vi "Compile Res Sim.vi"(8 "error in (no error)":errorcluster, 10 "SLSC Compiled in":T1 {"FIU Engine Data"."Ordered Fault Channels" format="%.0x"; "FIU Engine Data"."FIU IDs"."Slot #" max=15; "FIU Engine Data"."FIU IDs"."Chip Address (A2 A1 A0)" max=7}, 11 "Device Item Ref in":T7 format="%.0x") -> (0 "error out":errorcluster, 2 "SLSC Compiled out":T1 {"FIU Engine Data"."Ordered Fault Channels" format="%.0x"; "FIU Engine Data"."FIU IDs"."Slot #" max=15; "FIU Engine Data"."FIU IDs"."Chip Address (A2 A1 A0)" max=7}, 3 "Device Item Ref out":T7 format="%.0x")   [LabVIEW 2014, in "SLSC configuration System Explorer.lvlib"]
uses:
  SLSC configuration System Explorer.lvlib
  <vilib>/NI Veristand/Custom Device API/Custom Device Item Ref.ctl
  Shared/SLSC compiled.ctl
  Shared/Res Sim compiled.ctl
  Shared/Type Defs/FIU Engine Data.ctl
  Shared/Type Defs/FIU IDs.ctl
  Example/SPI Utility/Slot #.ctl
  Example/MCP23S17/Chip Address.ctl
  Shared/Card Postion.ctl
  <vilib>/NI Veristand/Custom Device API/Data Access Type.ctl
  Shared/Constants.vi
  <vilib>/NI Veristand/Custom Device API/Get Item Property (Variant).vi
  <vilib>/NI Veristand/Custom Device API/Get Item Property (U16).vi
  <vilib>/NI Veristand/Custom Device Tools/Custom Device Utility Library/Custom Device Utility Library.lvlib
  Shared/SLSC configuration Shared.lvlib
  <vilib>/NI Veristand/Custom Device API/Custom Device API.lvlib
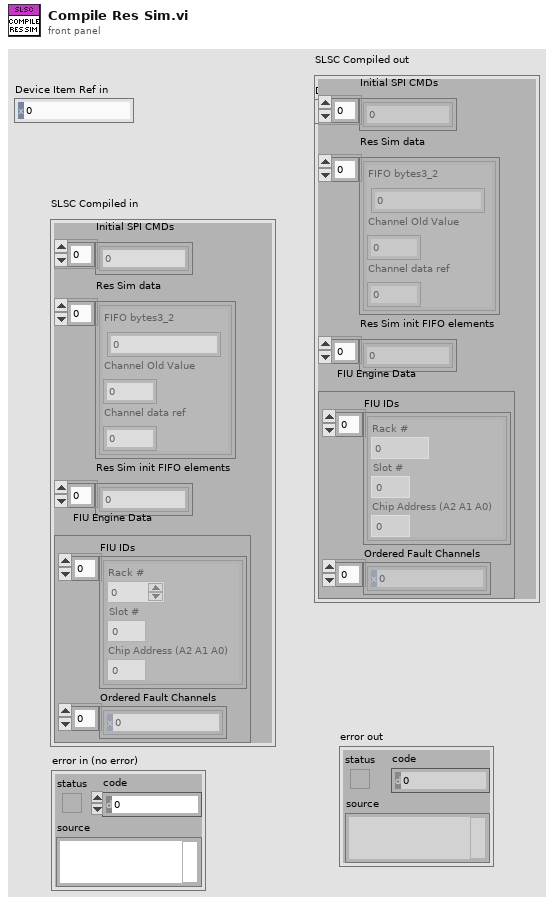
[diagram p1: front panel]
types:
  T1 = typedef "SLSC configuration Shared.lvlib/SLSC compiled.ctl" = cluster{"Initial SPI CMDs":u64[], "Res Sim data ":T2[], "Res Sim init FIFO elements":u32[], "FIU Engine Data":T3}
  T2 = typedef "SLSC configuration Shared.lvlib/Res Sim compiled.ctl" = cluster{"FIFO bytes3_2":u16, "Channel Old Value":dbl, "Channel data ref":i32}
  T3 = typedef "SLSC configuration Shared.lvlib/FIU Engine Data.ctl" = cluster{"FIU IDs":T4[], "Ordered Fault Channels":T7[]}
  T4 = typedef "SLSC configuration Shared.lvlib/FIU IDs.ctl" = cluster{"Rack #":u8, "Slot #":T5, "Chip Address (A2 A1 A0)":T6}
  T5 = typedef "SLSC configuration Shared.lvlib/Slot #.ctl" = u8
  T6 = typedef "SLSC configuration Shared.lvlib/Chip Address.ctl" = u8
  T7 = typedef "Custom Device API.lvlib/Custom Device Item Ref.ctl" = u64
  T8 = typedef "SLSC configuration Shared.lvlib/Card Postion.ctl" = cluster{"Chassis #":u8, "Slot #":u8}
  T9 = typedef "Custom Device API.lvlib/Data Access Type.ctl" = enum16{"Read", "Write"}
  T10 = typedef "Custom Device API.lvlib/Custom Device Channel.ctl" = cluster{"Type":T11, "Units":string, "Default Value":dbl, "Faultable":bool, "Scalable":bool}
  T11 = typedef "Custom Device API.lvlib/Custom Device Channel Type.ctl" = enum16{"Input", "Output"}
  T12 = typedef "Custom Device API.lvlib/Data Reference.ctl" = i32
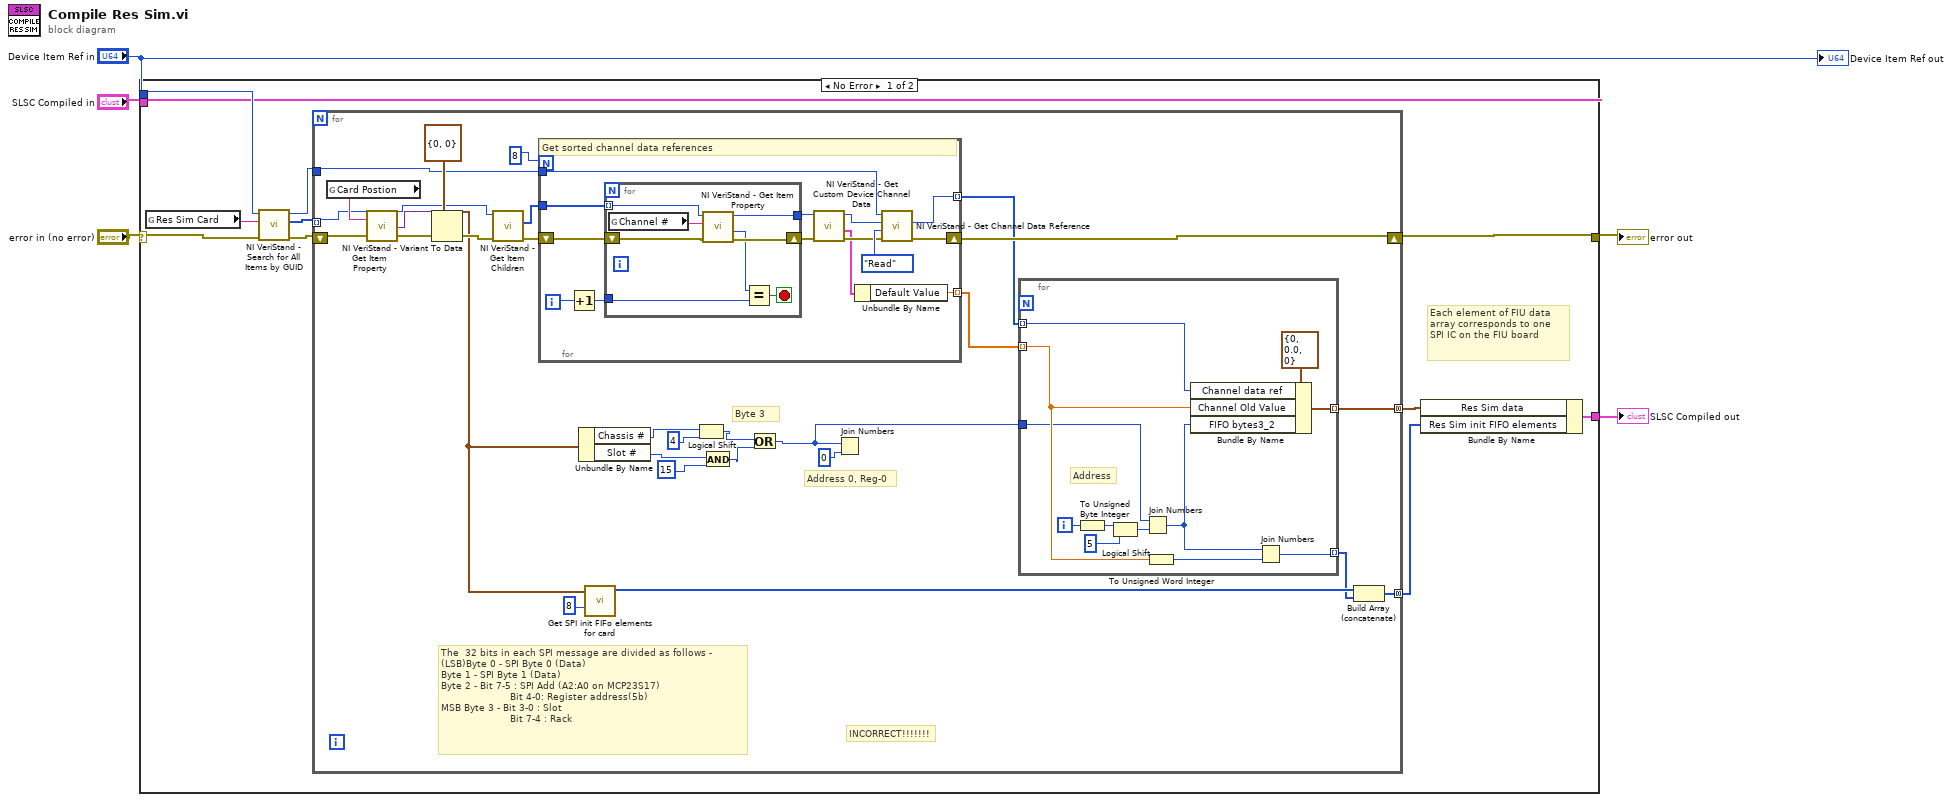
[diagram p0: block diagram]
diagram:
  n1 = case shown="No Error" "error in (no error)" {
    selector: "error in (no error)" -> [w9 w81]
    tunnel: [w12 w81] -> w5
    tunnel: "Device Item Ref in" -> [w11 _]
    tunnel: [w10 w80] -> w3
    tunnel: "SLSC Compiled in" -> [w8 w80]
    frame No Error {
      # "Each element of FIU data array corresponds to one SPI IC on the FIU board"
      n2 = global read "Constants.vi" "Res Sim Card"() -> (w16:string)
      n3 = call <vilib>:"NI VeriStand - Search for All Items by GUID.vi"("error in"=w9, "Item GUID"=w16, "Section Ref in"=w11) -> ("error out"=w15:errorcluster, "Item Refs"=w13:T7[], "Section Ref out"=w14:T7)  [unwired: 5 in, 1 out]
      n4 = for {
        tunnel: w14 -> [w29]
        tunnel: w13 -> [w31] mode=indexing
        tunnel: [w22] -> w7 mode=concatenating
        shift-right: [w24] -> w12
        shift-left: w15 -> [w39]
        tunnel: [w21] -> w6 mode=concatenating
        # "INCORRECT!!!!!!!"
        # "The  32 bits in each SPI message are divided as follows -\n(LSB)Byte 0 - SPI Byte 0 (Data)\nByte 1 - SPI Byte 1 (Data)\nByte 2 - Bit 7-5 : SPI Add (A2:A0 on MCP23S17)\n                       Bit 4-0: Register address(5b)\nMSB Byte 3 - Bit 3-0 : Slot\n                       Bit 7-4 : Rack"
        # "Address 0, Reg-0"
        # "Byte 3"
        n5 = global read "Constants.vi" "Card Postion"() -> (w38:string)
        n6 = call-poly <vilib>:"NI VeriStand - Get Item Property.vi"("error in (no error)"=w39, "Property Name"=w38, "Item Ref in"=w31) -> ("error out"=w41:errorcluster, "Value"=w42:variant, "Item Ref out"=w30:T7)  [unwired: 5 in, 1 out]
        n7 = Variant To Data(error in=w41, type=T8 {"Chassis #"=0, "Slot #"=0} ("Card Position"), Variant=w42) -> (data=w28:T8, error out=w40:errorcluster)
        n8 = call <vilib>:"NI VeriStand - Get Item Children.vi"("error in (no error)"=w40, "Item Ref in"=w30) -> ("error out"=w25:errorcluster, "Child Refs"=w44:T7[])  [unwired: 6 in, 2 out]
        n9 = for {
          N: 8 -> [_]
          tunnel: w44 -> [w70]
          tunnel: w29 -> [w68]
          tunnel: [w61] -> w19 mode=indexing
          tunnel: [w60] -> w20 mode=indexing
          shift-right: [w59] -> w24
          shift-left: w25 -> [w58]
          i -> [w71]
          # "Get sorted channel data references"
          n10 = Increment(x=w71) -> (x+1=w66:i32)
          n11 = for {
            shift-right: [w78] -> w69
            shift-left: w58 -> [w79]
            tunnel: w66 -> [w74]
            tunnel: w70 -> [w76] mode=indexing
            tunnel: [w72] -> w64
            stop <- w73 stop-if-true
            n12 = global read "Constants.vi" "Channel #"() -> (w77:string)
            n13 = call-poly <vilib>:"NI VeriStand - Get Item Property.vi"("error in (no error)"=w79, "Property Name"=w77, "Item Ref in"=w76) -> ("error out"=w78:errorcluster, "Value"=w75:u16, "Item Ref out"=w72:T7)  [unwired: 5 in, 1 out]
            n14 = Equal?(x=w75, y=w74) -> (x = y?=w73:bool)
          }
          n15 = call <vilib>:"NI VeriStand - Get Custom Device Channel Data.vi"("error in (no error)"=w69, "Channel Ref in"=w64) -> ("error out"=w65:errorcluster, "Channel"=w62:T10, "Channel Ref out"=w63:T7)  [unwired: 4 in, 3 out]
          n16 = Unbundle By Name(w62) -> ("Default Value"=w60:dbl)
          n17 = call <vilib>:"NI VeriStand - Get Channel Data Reference.vi"("error in (no error)"=w65, "Access"=Data_Access_Type."Read", "Channel Ref in"=w63, "Device Ref in"=w68) -> ("error out"=w59:errorcluster, "Channel Data Reference"=w61:T12)  [unwired: 5 in, 1 out]
        }
        n18 = Unbundle By Name(w28) -> ("Chassis #"=w37:u8, "Slot #"=w35:u8)
        n19 = call "Get SPI init FIFo elements for card.vi"("Num of SPI ICs"=u8 8, "Card Position"=w28) -> ("init FIFO elements"=w23:u32[])  [unwired: 9 in]
        n20 = Logical Shift(y=w37, x=u8 4) -> (x << y=w33:u8)
        n21 = And(x=w35, y=u8 15) -> (x .and. y?=w32:u8)
        n22 = Or(x=w33, y=w32) -> (x .or. y?=w18:u8)
        n23 = Join Numbers(hi=u8 0 ("lo"), lo=w18) -> ()  [unwired: 1 out]
        n24 = for {
          tunnel: [w55] -> w21 mode=indexing
          tunnel: w20 -> [w53] mode=indexing
          tunnel: w19 -> [w54] mode=indexing
          tunnel: w18 -> [w49]
          tunnel: [w46] -> w17 mode=indexing
          i -> [w52]
          # "Address"
          n25 = To Unsigned Byte Integer(number=w52) -> (unsigned 8bit integer=w51:u8)
          n26 = Logical Shift(y=w51, x=u8 5) -> (x << y=w48:u8)
          n27 = Join Numbers(hi=w49, lo=w48) -> ((hi.lo)=w47:u16)
          n28 = To Unsigned Word Integer(number=w53) -> (unsigned 16bit integer=w50:u16)
          n29 = Bundle By Name(cluster=T2 {"FIFO bytes3_2"=0, "Channel Old Value"=0.0, "Channel data ref"=0} ("Res Sim SPI command"), "Channel data ref"=w54, "Channel Old Value"=w53, "FIFO bytes3_2"=w47) -> (w55:T2)
          n30 = Join Numbers(hi=w47, lo=w50) -> ((hi.lo)=w46:u32)
        }
        n31 = Build Array (concatenate)(w23, w17) -> (w22:u32[])
      }
      n32 = Bundle By Name(cluster=w8, "Res Sim data"=w6, "Res Sim init FIFO elements"=w7) -> (w10:T1)
    }
    frame Error {
    }
  }
  "error out" <- w5
  "SLSC Compiled out" <- w3
  "Device Item Ref out" <- "Device Item Ref in"
